vi "Test Communication - 1.vi"() -> ()   [LabVIEW 2025]
uses:
  f24cd2ec-823b-4f95-a374-4134a1dae946.vi
  362e8ed5-b5fe-4805-bc07-5d5cfe9ff187.vi
  c76493dc-2eb4-4e37-bcd2-fc06ee71f938.vi
  523c6d7b-34c9-4a1f-add0-cf9b8ecace1d.vi
  a9163a1a-bf7f-4ec5-a553-ba6517dc0e79.vi
  6f03f4ed-4b4c-4e8a-979c-720ab53ff51f.vi
  PCAN2023/PCAN API.lvlib
  PCAN2023/PCAN2023/PCAN2023.lvlib
  77574cea-78a9-48c4-8703-67bd64e21fec.vi
panel:
  in  "x":bool
  out "Numeric":i32
  out "MessageBuffer out 2":T1 {"ID" format="%.0x"}
  out "Boolean 2":bool
  out "Boolean":bool
  out "MessageBuffer out":T1 {"ID" format="%.0x"}
  out "error out":errorcluster
  in  "error in":errorcluster
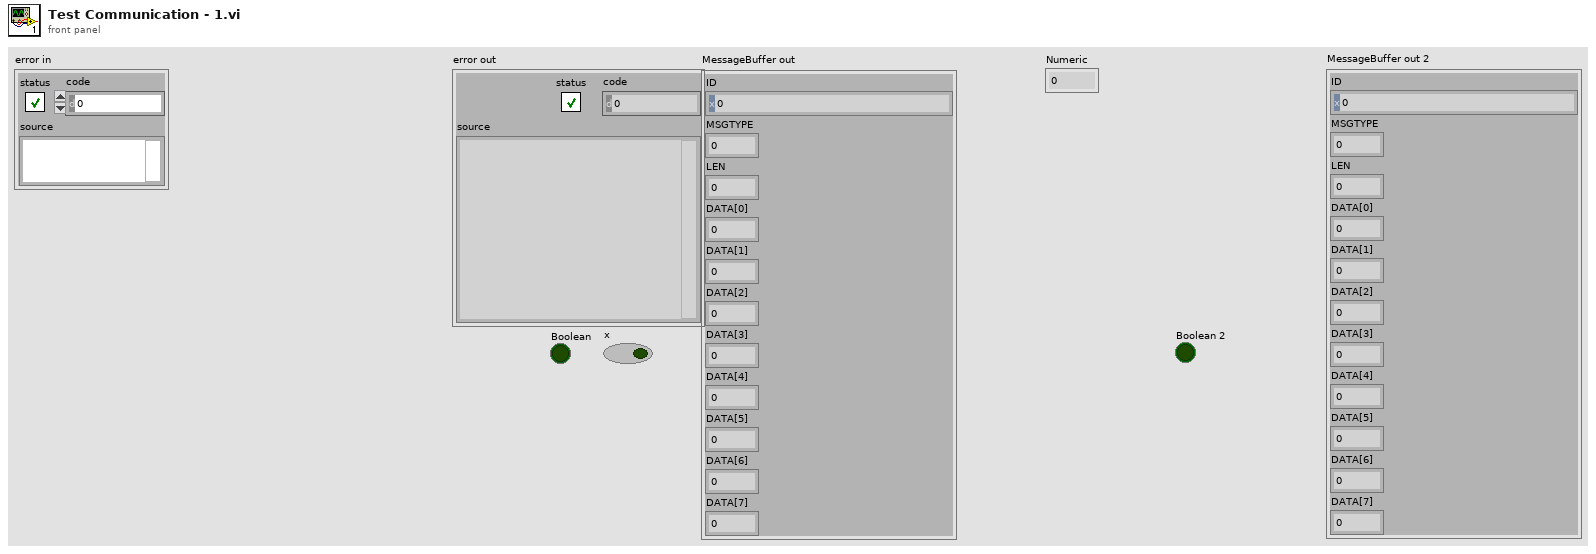
[diagram p1: front panel]
types:
  T1 = cluster{"ID":u32, "MSGTYPE":u8, "LEN":u8, "DATA[0]":u8, "DATA[1]":u8, "DATA[2]":u8, "DATA[3]":u8, "DATA[4]":u8, "DATA[5]":u8, "DATA[6]":u8, "DATA[7]":u8}
  T2 = cluster{"ID":u32, "MSGTYPE":u8, "DLC":u8, "DATA[0]":u8, "DATA[1]":u8, "DATA[2]":u8, "DATA[3]":u8, "DATA[4]":u8, "DATA[5]":u8, "DATA[6]":u8, "DATA[7]":u8, "DATA[8]":u8, "DATA[9]":u8, "DATA[10]":u8, "DATA[11]":u8, "DATA[12]":u8, "DATA[13]":u8, "DATA[14]":u8, "DATA[15]":u8, "DATA[16]":u8, "DATA[17]":u8, "DATA[18]":u8, "DATA[19]":u8, "DATA[20]":u8, "DATA[21]":u8, "DATA[22]":u8, "DATA[23]":u8, "DATA[24]":u8, "DATA[25]":u8, "DATA[26]":u8, "DATA[27]":u8, "DATA[28]":u8, "DATA[29]":u8, "DATA[30]":u8, "DATA[31]":u8, "DATA[32]":u8, "DATA[33]":u8, "DATA[34]":u8, "DATA[35]":u8, "DATA[36]":u8, "DATA[37]":u8, "DATA[38]":u8, "DATA[39]":u8, "DATA[40]":u8, "DATA[41]":u8, "DATA[42]":u8, "DATA[43]":u8, "DATA[44]":u8, "DATA[45]":u8, "DATA[46]":u8, "DATA[47]":u8, "DATA[48]":u8, "DATA[49]":u8, "DATA[50]":u8, "DATA[51]":u8, "DATA[52]":u8, "DATA[53]":u8, "DATA[54]":u8, "DATA[55]":u8, "DATA[56]":u8, "DATA[57]":u8, "DATA[58]":u8, "DATA[59]":u8, "DATA[60]":u8, "DATA[61]":u8, "DATA[62]":u8, "DATA[63]":u8}
  T3 = cluster{"ID":u32, "MSGTYPE":u8, "LEN":u8, "DATA[0]":u8, "DATA[1]":u8, "DATA[2]":u8, "DATA[3]":u8, "DATA[4]":u8, "DATA[5]":u8, "DATA[6]":u8, "DATA[7]":u8}[]
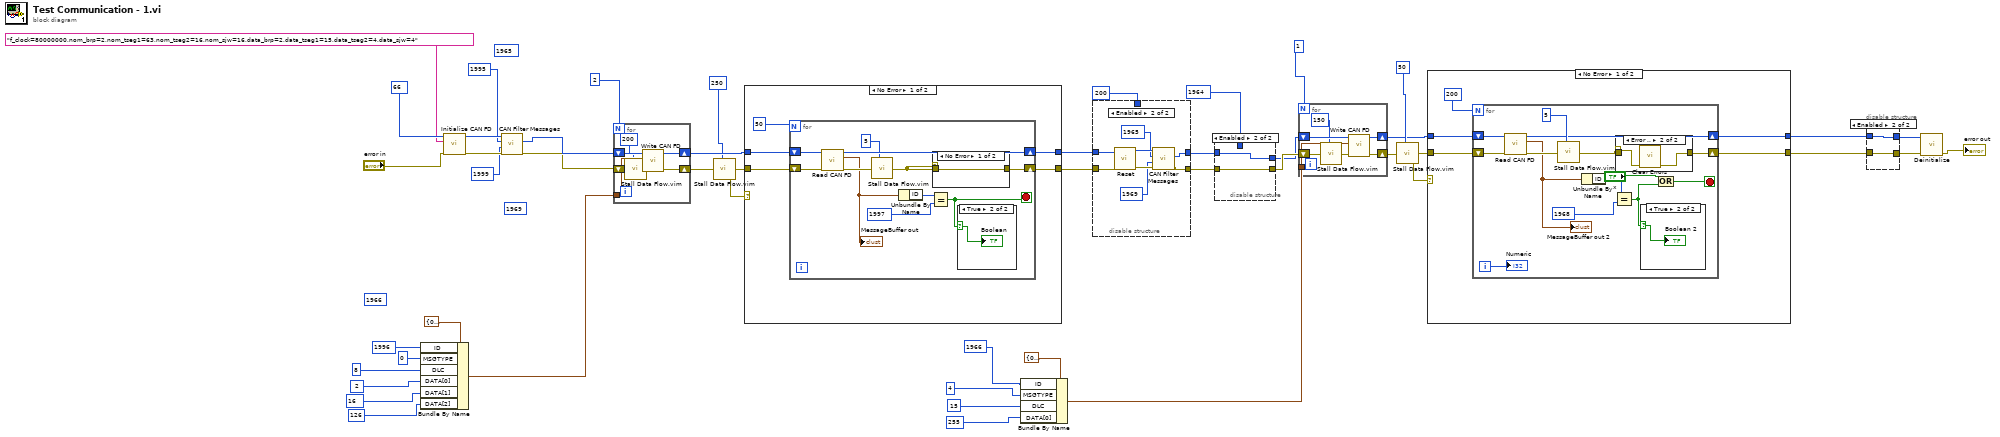
[diagram p0: block diagram]
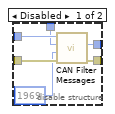
[diagram p2: hidden frame]
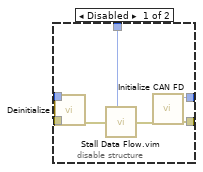
[diagram p3: hidden frame]
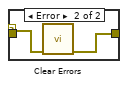
[diagram p4: hidden frame]
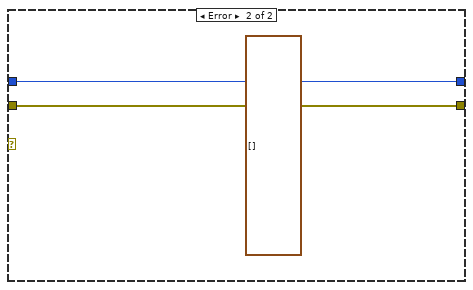
[diagram p6: hidden frame]
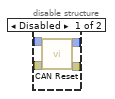
[diagram p7: hidden frame]
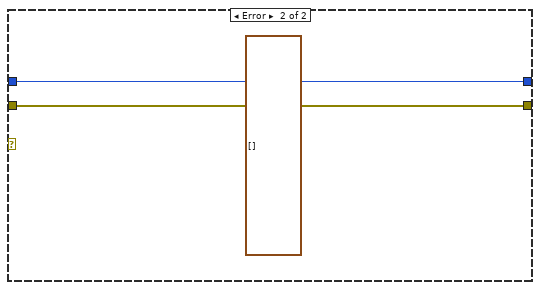
[diagram p10: hidden frame]
diagram:
  (unwired) u32 1969 ("FromID")
  (unwired) u32 1965 ("FromID")
  (unwired) u32 1966 ("ID")
  n1 = Bundle By Name(cluster=T2 {"ID"=0, "MSGTYPE"=0, "DLC"=0, "DATA[0]"=0, "DATA[1]"=0, "DATA[2]"=0, "DATA[3]"=0, "DATA[4]"=0, "DATA[5]"=0, "DATA[6]"=0, "DATA[7]"=0, "DATA[8]"=0, "DATA[9]"=0, "DATA[10]"=0, "DATA[11]"=0, "DATA[12]"=0, "DATA[13]"=0, "DATA[14]"=0, "DATA[15]"=0, "DATA[16]"=0, "DATA[17]"=0, "DATA[18]"=0, "DATA[19]"=0, "DATA[20]"=0, "DATA[21]"=0, "DATA[22]"=0, "DATA[23]"=0, "DATA[24]"=0, "DATA[25]"=0, "DATA[26]"=0, "DATA[27]"=0, "DATA[28]"=0, "DATA[29]"=0, "DATA[30]"=0, "DATA[31]"=0, "DATA[32]"=0, "DATA[33]"=0, "DATA[34]"=0, "DATA[35]"=0, "DATA[36]"=0, "DATA[37]"=0, "DATA[38]"=0, "DATA[39]"=0, "DATA[40]"=0, "DATA[41]"=0, "DATA[42]"=0, "DATA[43]"=0, "DATA[44]"=0, "DATA[45]"=0, "DATA[46]"=0, "DATA[47]"=0, "DATA[48]"=0, "DATA[49]"=0, "DATA[50]"=0, "DATA[51]"=0, "DATA[52]"=0, "DATA[53]"=0, "DATA[54]"=0, "DATA[55]"=0, "DATA[56]"=0, "DATA[57]"=0, "DATA[58]"=0, "DATA[59]"=0, "DATA[60]"=0, "DATA[61]"=0, "DATA[62]"=0, "DATA[63]"=0} ("MessageBuffer"), "ID"=u32 1996, "MSGTYPE"=u8 0, "DLC"=u8 8, "DATA[0]"=u8 2, "DATA[1]"=u8 16 ("DATA[0]"), "DATA[2]"=u8 126 ("DATA[0]")) -> (w42:T2)
  n2 = call "Initialize CAN FD.vi"("error in"="error in", "BitrateFD"="f_clock=80000000,nom_brp=2,nom_tseg1=63,nom_tseg2=16,nom_sjw=16,data_brp=2,data_tseg1=15,data_tseg2=4,data_sjw=4", "Channel"=u16 66) -> ("error out"=w35:errorcluster, "Channel out"=w36:u16)  [unwired: 7 in]
  n3 = call "CAN Filter Messages.vi"("error in (no error)"=w35, "ToID"=u32 1999 ("FromID"), "FromID"=u32 1995, "Channel"=w36) -> ("error out"=w14:errorcluster, "Channel out"=w15:u16)  [unwired: 5 in, 1 out]
  n4 = for {
    N: 2 -> [_]
    tunnel: w42 -> [w51]
    shift-right: [w50] -> w13
    shift-left: w15 -> [w53]
    shift-right: [w49] -> w12
    shift-left: w14 -> [w52]
    n5 = call "Stall Data Flow.vim"("value in"=w52, "milliseconds to wait"=u32 200) -> ("value out"=w48:errorcluster)  [unwired: 1 out]
    n6 = call "Write CAN FD.vi"("error in (no error)"=w48, "MessageBuffer"=w51, "Channel"=w53) -> ("error out"=w49:errorcluster, "Channel out"=w50:u16)  [unwired: 7 in]
  }
  n7 = call "Stall Data Flow.vim"("value in"=w12, "milliseconds to wait"=u32 250) -> ("value out"=w10:errorcluster)  [unwired: 1 out]
  n8 = case shown="No Error" w10 {
    tunnel: w13 -> [w58 w75]
    tunnel: w10 -> [w57 w74]
    tunnel: [w56 w75] -> w8
    tunnel: [w55 w74] -> w7
    frame No Error {
      n9 = for {
        N: 50 -> [_]
        shift-right: [w65] -> w56
        shift-left: w58 -> [w66]
        shift-right: [w67] -> w55
        shift-left: w57 -> [w64]
        stop <- w61 stop-if-true
        n10 = call "Read CAN FD.vi"("error in"=w64, "Channel"=w66) -> ("error out"=w63:errorcluster, "MessageBuffer out"=w62:T1, "Channel out"=w65:u16)  [unwired: 7 in]
        "MessageBuffer out" <- w62
        n11 = call "Stall Data Flow.vim"("value in"=w63, "milliseconds to wait"=u32 5) -> ("value out"=w60:errorcluster)  [unwired: 1 out]
        n12 = Unbundle By Name(w62) -> ("ID"=w69:u32)
        n13 = Equal?(x=w69, y=u32 1997) -> (x = y?=w61:bool)
        n14 = case shown="No Error" w60 {
          selector: w60 -> [w70 w72]
          tunnel: w60 -> [_ _]
          tunnel: [w70 w71] -> w67
          frame No Error {
          }
          frame Error {
            n15 = call <vilib>:"Clear Errors.vi"("error in (no error)"=w72) -> ("error out"=w71:errorcluster)  [unwired: 5 in, 1 out]
          }
        }
        n16 = case shown="True" w61 {
          selector: w61 -> [_ w73]
          frame False {
          }
          frame True {
            "Boolean" <- w73
          }
        }
      }
    }
    frame Error {
      (unwired) T3 []
    }
  }
  n17 = Bundle By Name(cluster=T2 {"ID"=0, "MSGTYPE"=0, "DLC"=0, "DATA[0]"=0, "DATA[1]"=0, "DATA[2]"=0, "DATA[3]"=0, "DATA[4]"=0, "DATA[5]"=0, "DATA[6]"=0, "DATA[7]"=0, "DATA[8]"=0, "DATA[9]"=0, "DATA[10]"=0, "DATA[11]"=0, "DATA[12]"=0, "DATA[13]"=0, "DATA[14]"=0, "DATA[15]"=0, "DATA[16]"=0, "DATA[17]"=0, "DATA[18]"=0, "DATA[19]"=0, "DATA[20]"=0, "DATA[21]"=0, "DATA[22]"=0, "DATA[23]"=0, "DATA[24]"=0, "DATA[25]"=0, "DATA[26]"=0, "DATA[27]"=0, "DATA[28]"=0, "DATA[29]"=0, "DATA[30]"=0, "DATA[31]"=0, "DATA[32]"=0, "DATA[33]"=0, "DATA[34]"=0, "DATA[35]"=0, "DATA[36]"=0, "DATA[37]"=0, "DATA[38]"=0, "DATA[39]"=0, "DATA[40]"=0, "DATA[41]"=0, "DATA[42]"=0, "DATA[43]"=0, "DATA[44]"=0, "DATA[45]"=0, "DATA[46]"=0, "DATA[47]"=0, "DATA[48]"=0, "DATA[49]"=0, "DATA[50]"=0, "DATA[51]"=0, "DATA[52]"=0, "DATA[53]"=0, "DATA[54]"=0, "DATA[55]"=0, "DATA[56]"=0, "DATA[57]"=0, "DATA[58]"=0, "DATA[59]"=0, "DATA[60]"=0, "DATA[61]"=0, "DATA[62]"=0, "DATA[63]"=0} ("MessageBuffer"), "ID"=u32 1966, "MSGTYPE"=u8 4, "DLC"=u8 15, "DATA[0]"=u8 255) -> (w28:T2)
  n18 = disable-structure shown="Enabled" {
    disable-tunnel: w8 -> [w82 w90]
    disable-tunnel: w7 -> [w81 w89]
    disable-tunnel: [w80 w87] -> w6
    disable-tunnel: [w78 w85] -> w5
    disable-tunnel: u32 200 ("milliseconds to wait") -> [w76 _]
    frame Disabled {
      n19 = call "Deinitialize.vi"("error in"=w81, "Channel"=w82) -> ("error out"=w79:errorcluster)  [unwired: 9 in]
      n20 = call "Stall Data Flow.vim"("value in"=w79, "milliseconds to wait"=w76) -> ("value out"=w77:errorcluster)  [unwired: 1 out]
      n21 = call "Initialize CAN FD.vi"("error in"=w77) -> ("error out"=w78:errorcluster, "Channel out"=w80:u16)  [unwired: 9 in]
    }
    frame Enabled {
      n22 = call "Reset.vi"("error in"=w89, "Channel"=w90) -> ("error out"=w86:errorcluster, "Channel out"=w88:u16)  [unwired: 8 in]
      n23 = call "CAN Filter Messages.vi"("error in (no error)"=w86, "ToID"=u32 1969 ("FromID"), "FromID"=u32 1965, "Channel"=w88) -> ("error out"=w85:errorcluster, "Channel out"=w87:u16)  [unwired: 5 in, 1 out]
    }
  }
  n24 = disable-structure shown="Enabled" {
    disable-tunnel: w6 -> [w96 w97]
    disable-tunnel: w5 -> [w95 w98]
    disable-tunnel: [w94 w98] -> w4
    disable-tunnel: [w93 w97] -> w3
    disable-tunnel: u32 1964 ("FromID") -> [w92 _]
    frame Disabled {
      n25 = call "CAN Filter Messages.vi"("error in (no error)"=w95, "ToID"=u32 1969 ("FromID"), "FromID"=w92, "Channel"=w96) -> ("error out"=w94:errorcluster, "Channel out"=w93:u16)  [unwired: 5 in, 1 out]
    }
    frame Enabled {
    }
  }
  n26 = for {
    N: 1 -> [_]
    tunnel: w28 -> [w103]
    shift-right: [w102] -> w25
    shift-left: w3 -> [w105]
    shift-right: [w101] -> w24
    shift-left: w4 -> [w104]
    n27 = call "Stall Data Flow.vim"("value in"=w104, "milliseconds to wait"=u32 150) -> ("value out"=w100:errorcluster)  [unwired: 1 out]
    n28 = call "Write CAN FD.vi"("error in (no error)"=w100, "MessageBuffer"=w103, "Channel"=w105) -> ("error out"=w101:errorcluster, "Channel out"=w102:u16)  [unwired: 7 in]
  }
  n29 = call "Stall Data Flow.vim"("value in"=w24, "milliseconds to wait"=u32 50) -> ("value out"=w26:errorcluster)  [unwired: 1 out]
  n30 = case shown="No Error" w26 {
    tunnel: w25 -> [w110 w130]
    tunnel: w26 -> [w109 w129]
    tunnel: [w108 w130] -> w23
    tunnel: [w107 w129] -> w21
    frame No Error {
      n31 = for {
        N: 200 -> [_]
        shift-right: [w119] -> w108
        shift-left: w110 -> [w120]
        shift-right: [w122] -> w107
        shift-left: w109 -> [w118]
        i -> [w115]
        stop <- w112 stop-if-true
        n32 = call "Read CAN FD.vi"("error in"=w118, "Channel"=w120) -> ("error out"=w117:errorcluster, "MessageBuffer out"=w111:T1, "Channel out"=w119:u16)  [unwired: 7 in]
        "MessageBuffer out 2" <- w111
        n33 = call "Stall Data Flow.vim"("value in"=w117, "milliseconds to wait"=u32 5) -> ("value out"=w121:errorcluster)  [unwired: 1 out]
        n34 = Unbundle By Name(w111) -> ("ID"=w116:u32)
        n35 = Equal?(x=w116, y=u32 1968) -> (x = y?=w114:bool)
        n36 = case shown="Error .." w121 {
          selector: w121 -> [w125 w127]
          tunnel: w121 -> [_ _]
          tunnel: [w125 w126] -> w122
          frame No Error {
          }
          frame Error {
            n37 = call <vilib>:"Clear Errors.vi"("error in (no error)"=w127) -> ("error out"=w126:errorcluster)  [unwired: 5 in, 1 out]
          }
        }
        n38 = case shown="True" w114 {
          selector: w114 -> [_ w128]
          frame False {
          }
          frame True {
            "Boolean 2" <- w128
          }
        }
        n39 = Or(x="x", y=w114) -> (x .or. y?=w112:bool)
        "Numeric" <- w115
      }
    }
    frame Error {
      (unwired) T3 []
    }
  }
  n40 = disable-structure shown="Enabled" {
    disable-tunnel: w23 -> [w134 w136]
    disable-tunnel: [w133 w136] -> w22
    disable-tunnel: [w132 w135] -> w20
    disable-tunnel: w21 -> [w131 w135]
    frame Disabled {
      n41 = call "CAN Reset.vi"("error in"=w131, "Channel"=w134) -> ("error out"=w132:errorcluster, "Channel out"=w133:u16)  [unwired: 7 in, 1 out]
    }
    frame Enabled {
    }
  }
  n42 = call "Deinitialize.vi"("error in"=w20, "Channel"=w22) -> ("error out"=→"error out":errorcluster)  [unwired: 9 in]
